vi "DSF.Engine.Plugin.Sort by Priority.vi"(8 "error in (no error)":errorcluster, 11 "Plugins in":refnum<class "DSF.Engine.Plugin.lvclass">[](array[class])) -> (0 "error out":errorcluster, 3 "Plugins out":refnum<class "DSF.Engine.Plugin.lvclass">[](array[class]))   [LabVIEW 2017, in "DSF.Engine.lvlib" / "DSF.Engine.Plugin.lvclass"]
uses:
  DSF.Engine.Plugin.lvclass
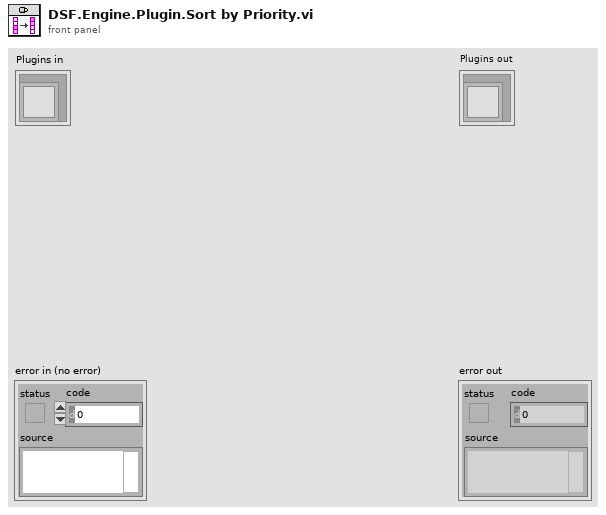
[diagram p1: front panel]
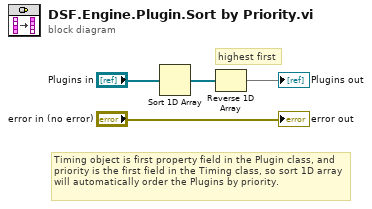
[diagram p0: block diagram]
diagram:
  # "Timing object is first property field in the Plugin class, and priority is the first field in the Timing class, so sort 1D array will automatically order the Plugins by priority."
  # "highest first"
  n1 = Sort 1D Array(array="Plugins in") -> (sorted array=w3:refnum<class "DSF.Engine.Plugin.lvclass">[])
  n2 = Reverse 1D Array(array=w3) -> (reversed array=→"Plugins out":refnum<class "DSF.Engine.Plugin.lvclass">[])
  "error out" <- "error in (no error)"
